vi "Go to Coordinate.vi"(7 "Description":string="Reserve", 8 "Command Info":T1, 11 "Coordinates":cluster{"X":dbl, "Y":dbl, "Angle":dbl}) -> (0 "Command Info":T1)   [LabVIEW 2015]
uses:
  <vilib>/Rock Robotics/WPI/Framework/Command Status Info.ctl
  <vilib>/Rock Robotics/WPI/Framework/Completion Status.ctl
  <vilib>/Rock Robotics/WPI/Framework/Completion Notifier.ctl
  Implementation/Swerve Drive Setpoints.ctl
  Implementation/Swerve Drive Operations.ctl
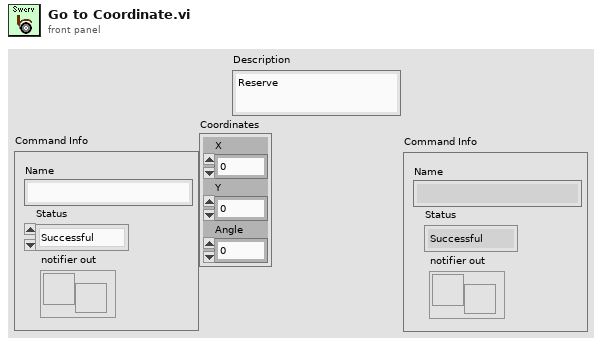
[diagram p1: front panel]
types:
  T1 = typedef "Command Status Info.ctl" = cluster{"Name":string, "Status":T2, "notifier out":T3}
  T2 = typedef "Completion Status.ctl" = enum16{"Successful", "Aborted", "Incomplete"}
  T3 = typedef "Completion Notifier.ctl" = refnum<notifier>
  T4 = typedef "Swerve Drive Setpoints.ctl" = cluster{"Operation":T5, "Duration":dbl, "Strafe Joystick Axes":cluster{"X":dbl, "Y":dbl}, "Face Joystick Axes":cluster{"X":dbl, "Y":dbl}, "Trigger Axes":cluster{"Left":dbl, "Right":dbl}, "Coordinates":cluster{"X":dbl, "Y":dbl, "Angle":dbl}}
  T5 = typedef "Swerve Drive Operations.ctl" = enum16{"Reserve", "Read Current", "Immediate", "Go to Coordinate", "Drive Immediate (Turn Speed/Face and Stafe)"}
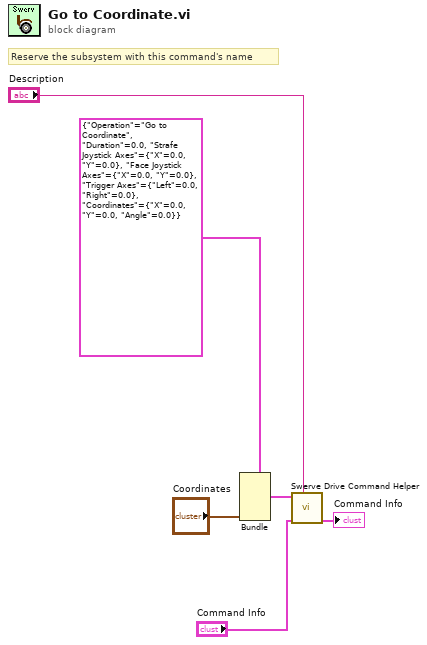
[diagram p0: block diagram]
diagram:
  # "Reserve the subsystem with this command's name"
  n1 = Bundle(cluster=T4 {"Operation"=enum."Go to Coordinate", "Duration"=0.0, "Strafe Joystick Axes"={"X"=0.0, "Y"=0.0}, "Face Joystick Axes"={"X"=0.0, "Y"=0.0}, "Trigger Axes"={"Left"=0.0, "Right"=0.0}, "Coordinates"={"X"=0.0, "Y"=0.0, "Angle"=0.0}} ("SubSystem Data"), "Coordinates"="Coordinates") -> (w2:T4)  [unwired: 5 in]
  n2 = call "Swerve Drive Command Helper.vi"("Description"="Description", "Command Info In"="Command Info", "SubSystem Data"=w2) -> ("Command Info Out"=→"Command Info":T1)  [unwired: 7 in, 1 out]
